vi "Test LoadCell200K_MBDC API.vi"() -> ()   [LabVIEW 2016]
doc: "LoadCell200K_MBDC API Tester."
uses:
  LoadCell200K_MBDC.lvlib
panel:
  in  "wait for reply":bool=TRUE
  in  "Show Block Diagram":bool
  in  "X":dbl=1.0
  out "Reply Payload":dbl
  in  "Stop Module":bool
  in  "Start Module":bool
  out "Do Something Count":i32
  in  "Test Do Something Else and Wait for Reply":bool
  in  "Hide Module Panel":bool
  in  "Show Module Panel":bool
  in  "Test Do Something Else":bool
  in  "Test Do Something":bool
  out "Status":string
  out "Module Running?":bool
  # "This VI tests the API for the Module."
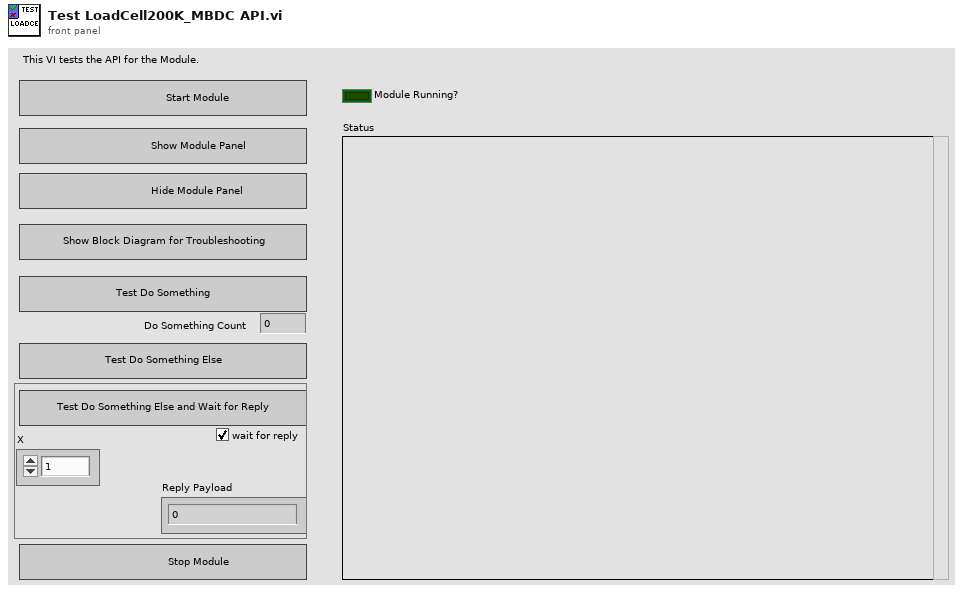
[diagram p1: front panel]
types:
  T1 = typedef "LoadCell200K_MBDC.lvlib/Broadcast Events--cluster.ctl" = cluster{"Module Did Init":refnum<user-event>, "Status Updated":refnum<user-event>, "Error Reported":refnum<user-event>, "Did Something":refnum<user-event>, "Module Did Stop":refnum<user-event>, "Update Module Execution Status":refnum<user-event>}
  T2 = typedef "LoadCell200K_MBDC.lvlib/Do Something Else and Wait (Reply Payload)--cluster.ctl" = cluster{"Value":dbl, "error":errorcluster}
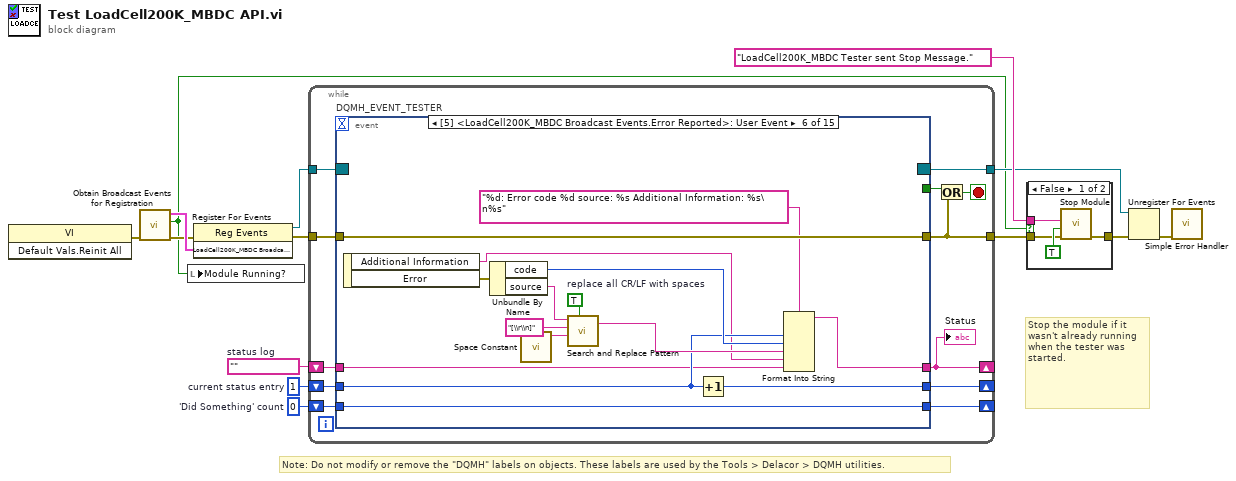
[diagram p0: block diagram]
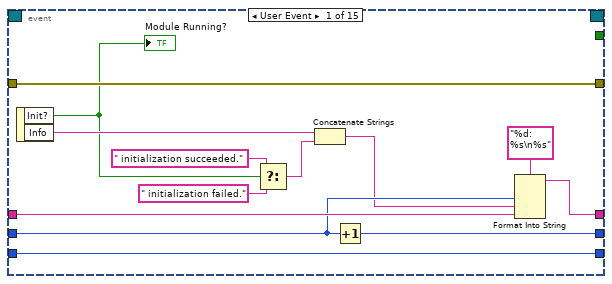
[diagram p3: hidden frame]
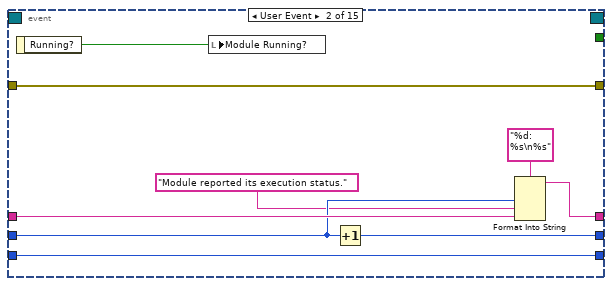
[diagram p4: hidden frame]
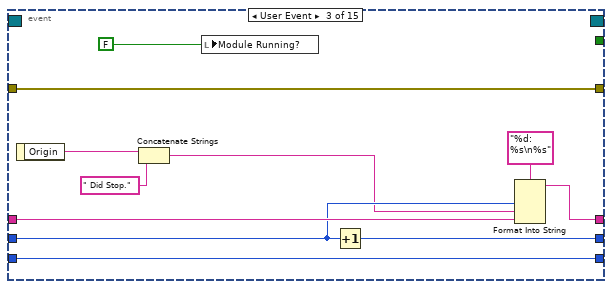
[diagram p5: hidden frame]
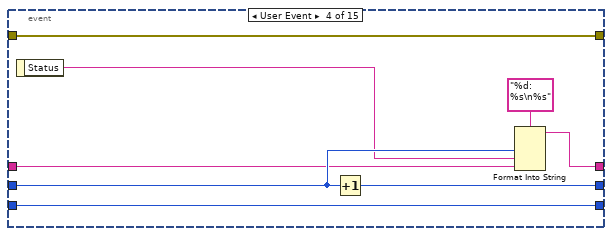
[diagram p6: hidden frame]
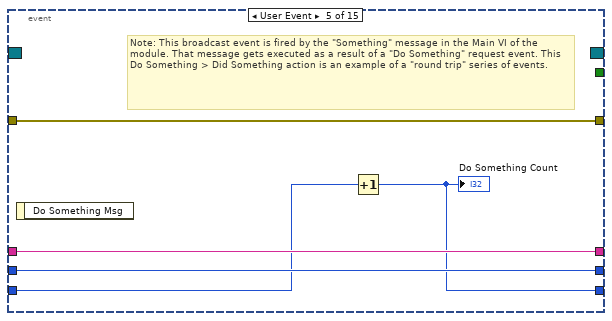
[diagram p7: hidden frame]
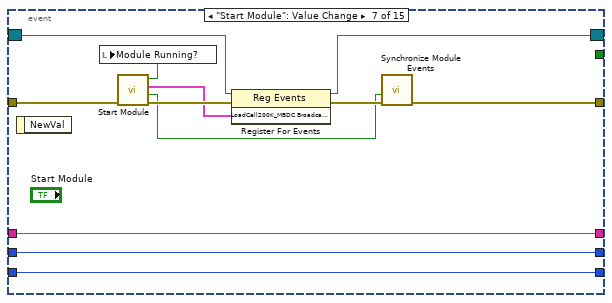
[diagram p8: hidden frame]
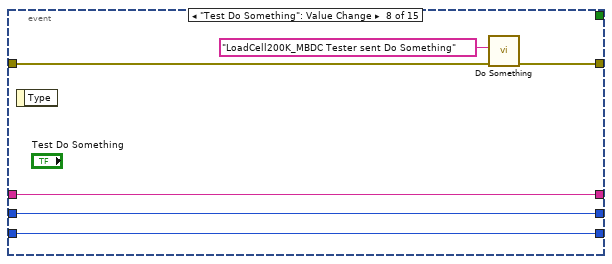
[diagram p9: hidden frame]
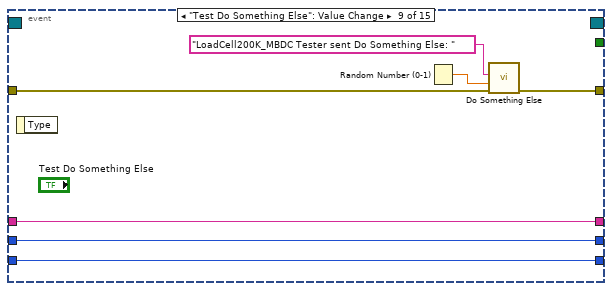
[diagram p10: hidden frame]
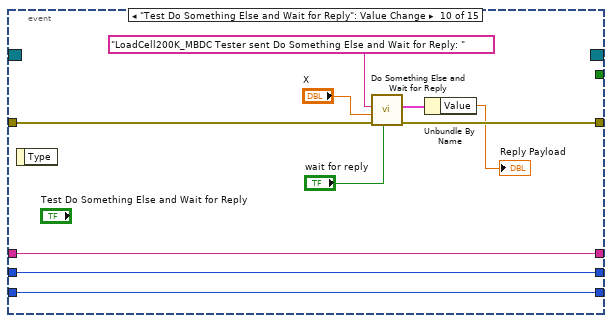
[diagram p11: hidden frame]
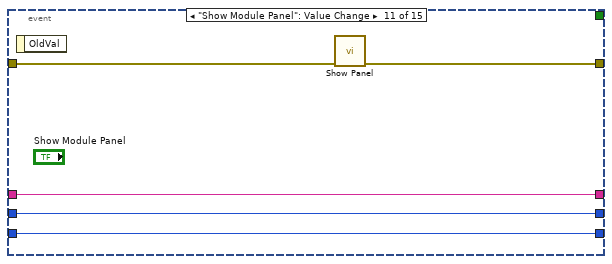
[diagram p12: hidden frame]
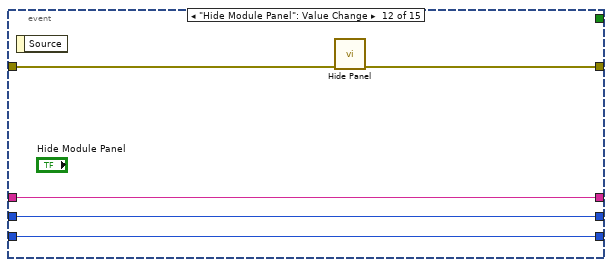
[diagram p13: hidden frame]
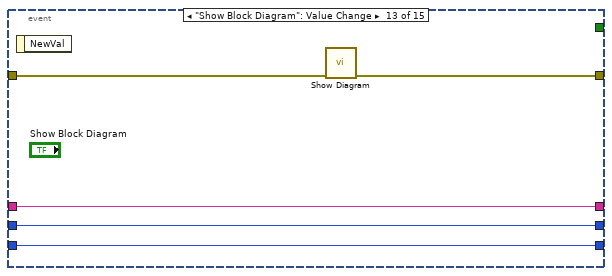
[diagram p14: hidden frame]
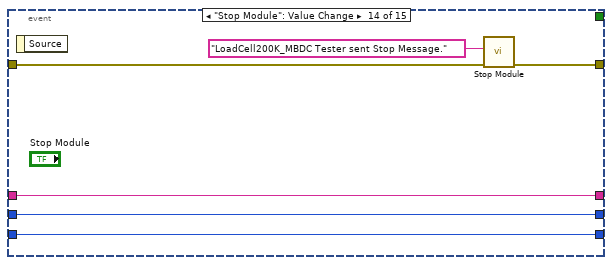
[diagram p15: hidden frame]
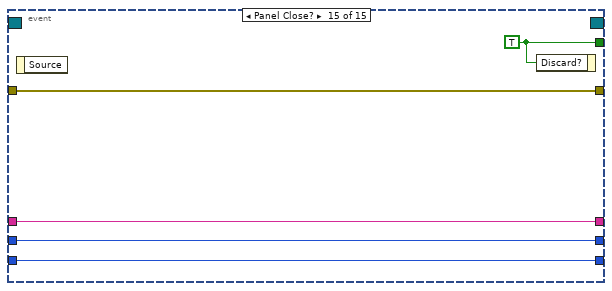
[diagram p16: hidden frame]
diagram:
  w10 = 0  # 'Did Something' count
  w11 = 1  # current status entry
  w12 = ""  # status log
  # "Stop the module if it wasn't already running when the tester was started."
  # "Note: Do not modify or remove the \"DQMH\" labels on objects. These labels are used by the Tools > Delacor > DQMH utilities."
  n1 = invoke class="VI" method="Default Vals.Reinit All"() -> (error out=w5:errorcluster)  [unwired: 3 in, 2 out]
  n2 = call "Obtain Broadcast Events for Registration.vi"("error in (no error)"=w5) -> ("error out"=w4:errorcluster, "Already running?"=w3:bool, "LoadCell200K_MBDC Broadcast Events"=w8:T1)  [unwired: 8 in]
  n3 = local write "Module Running?"(w3) -> ()
  n4 = register-events(error in=w4, w8) -> (reference out=w7:refnum<event-registration>, error out=w9:errorcluster)  [unwired: 1 in]
  n5 = while {
    tunnel: w7 -> [w26]
    tunnel: [w15] -> w2
    shift-right: [w21] -> _
    shift-left: w12 -> [w23]
    shift-right: [w22] -> _
    shift-left: w11 -> [w24]
    shift-right: [w19] -> _
    shift-left: w10 -> [w20]
    tunnel: w9 -> [w17]
    tunnel: [w16] -> w6
    stop <- w18 stop-if-true
    n6 = event "DQMH_EVENT_TESTER" shown="[5] <LoadCell200K_MBDC Broadcast Events.Error Reported>: User Event" {
      selector: w26 -> [_ _ _ _ _ _ w92 _ _ _ _ _ _ _ _]
      dyn-events: [_ _ _ _ _ _ w91 _ _ _ _ _ _ _ _] -> w16
      timeout: _ -> [_ _ _ _ _ _ _ _ _ _ _ _ _ _ _]
      tunnel: [_ _ _ _ _ _ _ _ _ _ _ _ _ _ w148] -> w25
      tunnel: [w39 w41 w49 w60 w68 w86 w90 w105 w112 w122 w127 w132 w133 w140 w144] -> w15
      tunnel: w24 -> [w36 w46 w57 w64 w71 w76 w96 w102 w108 w119 w125 w130 w135 w142 w146]
      tunnel: w23 -> [w37 w47 w58 w63 w72 w74 w97 w103 w109 w120 w126 w131 w136 w143 w147]
      tunnel: [w34 w44 w55 w65 w72 w77 w97 w103 w109 w120 w126 w131 w136 w143 w147] -> w21
      tunnel: [w35 w45 w56 w67 w71 w75 w96 w102 w108 w119 w125 w130 w135 w142 w146] -> w22
      tunnel: w20 -> [w31 w42 w51 w61 w70 w87 w95 w101 w107 w118 w124 w129 w134 w141 w145]
      tunnel: [w31 w42 w51 w61 w69 w87 w95 w101 w107 w118 w124 w129 w134 w141 w145] -> w19
      tunnel: w17 -> [w39 w41 w49 w60 w68 w86 w89 w100 w106 w115 w123 w128 w137 w138 w144]
      event User Event {
        n7 = event-data() -> ("Init?"=w30:bool, "Info"=w33:string)  [unwired: 1 in]
        "Module Running?" <- w30
        n8 = Select(t=" initialization succeeded.", s=w30, f=" initialization failed.") -> (s? t:f=w27:string)
        n9 = Concatenate Strings(w33, w27) -> (w32:string)
        n10 = Increment(x=w36) -> (x+1=w35:i32)
        n11 = Format Into String(format string="%d: %s\n%s", w36, w32, w37) -> (resulting string=w34:string)  [unwired: 2 in, 1 out]
      }
      event User Event {
        n12 = event-data() -> ("Running?"=w40:bool)  [unwired: 1 in]
        n13 = local write "Module Running?"(w40) -> ()
        n14 = Increment(x=w46) -> (x+1=w45:i32)
        n15 = Format Into String(format string="%d: %s\n%s", w46, "Module reported its execution status.", w47) -> (resulting string=w44:string)  [unwired: 2 in, 1 out]
      }
      event User Event {
        n16 = event-data() -> ("Origin"=w54:string)  [unwired: 1 in]
        n17 = Concatenate Strings(w54, " Did Stop.") -> (w53:string)
        n18 = local write "Module Running?"(FALSE ("Module Did Init?")) -> ()
        n19 = Increment(x=w57) -> (x+1=w56:i32)
        n20 = Format Into String(format string="%d: %s\n%s", w57, w53, w58) -> (resulting string=w55:string)  [unwired: 2 in, 1 out]
      }
      event User Event {
        n21 = event-data() -> ("Status"=w62:string)  [unwired: 1 in]
        n22 = Increment(x=w64) -> (x+1=w67:i32)
        n23 = Format Into String(format string="%d: %s\n%s", w64, w62, w63) -> (resulting string=w65:string)  [unwired: 2 in, 1 out]
      }
      event User Event {
        # "Note: This broadcast event is fired by the \"Something\" message in the Main VI of the module. That message gets executed as a result of a \"Do Something\" request event. This Do Something > Did Something action is an example of a \"round trip\" series of events."
        n24 = event-data() -> ()  [unwired: 1 in, 1 out]
        n25 = Increment(x=w70) -> (x+1=w69:i32)
        "Do Something Count" <- w69
      }
      event User Event {
        w82 = TRUE  # replace all CR/LF with spaces
        n26 = event-data() -> ("Additional Information"=w73:string, "Error"=w78:errorcluster)  [unwired: 1 in]
        n27 = Unbundle By Name(w78) -> ("code"=w79:i32, "source"=w80:string)
        n28 = call <vilib>:"Space Constant.vi"() -> ("String"=w83:string)
        n29 = call <vilib>:"Search and Replace Pattern.vi"("string"=w80, "regular expression (\"\")"="[\\r\\n]" ("regular expression (\"\")"), "replace string (\"\")"=w83, "replace all? (F)"=w82) -> ("result string"=w81:string)  [unwired: 1 in, 1 out]
        n30 = Increment(x=w76) -> (x+1=w75:i32)
        n31 = Format Into String(format string="%d: Error code %d source: %s Additional Information: %s\n%s", w76, w79, w81, w73, w74) -> (resulting string=w77:string)  [unwired: 2 in, 1 out]
      }
      event "Start Module": Value Change {
        n32 = event-data() -> ()  [unwired: 1 in, 1 out]
        n33 = call "Start Module.vi"("error in (no error)"=w89) -> ("error out"=w98:errorcluster, "Wait for Event Sync?"=w94:bool, "LoadCell200K_MBDC Broadcast Events"=w93:T1, "Module Was Already Running?"=w88:bool)  [unwired: 7 in]
        n34 = local write "Module Running?"(w88) -> ()
        n35 = register-events(reference=w92, error in=w98, w93) -> (reference out=w91:refnum<event-registration>, error out=w99:errorcluster)
        n36 = call "Synchronize Module Events.vi"("error in"=w99, "Wait for Event Sync?"=w94) -> ("error out"=w90:errorcluster)  [unwired: 9 in]
      }
      event "Test Do Something": Value Change {
        n37 = event-data() -> ()  [unwired: 1 in, 1 out]
        n38 = call "Do Something.vi"("error in (no error)"=w100, "Do Something Message"="LoadCell200K_MBDC Tester sent Do Something") -> ("error out"=w105:errorcluster)  [unwired: 9 in]
      }
      event "Test Do Something Else": Value Change {
        n39 = event-data() -> ()  [unwired: 1 in, 1 out]
        n40 = Random Number (0-1)() -> (number: 0 to 1=w110:dbl)
        n41 = call "Do Something Else.vi"("error in (no error)"=w106, "X"=w110, "Do Something Else Message"="LoadCell200K_MBDC Tester sent Do Something Else: " ("Do Something Message")) -> ("error out"=w112:errorcluster)  [unwired: 8 in]
      }
      event "Test Do Something Else and Wait for Reply": Value Change {
        n42 = event-data() -> ()  [unwired: 1 in, 1 out]
        n43 = call "Do Something Else and Wait for Reply.vi"("wait for reply (T)"="wait for reply", "error in (no error)"=w115, "X"="X", "Do Something Else Message"="LoadCell200K_MBDC Tester sent Do Something Else and Wait for Reply: " ("Do Something Message")) -> ("error out"=w122:errorcluster, "Reply Payload"=w117:T2)  [unwired: 5 in, 1 out]
        n44 = Unbundle By Name(w117) -> ("Value"=→"Reply Payload":dbl)
      }
      event "Show Module Panel": Value Change {
        n45 = event-data() -> ()  [unwired: 1 in, 1 out]
        n46 = call "Show Panel.vi"("error in (no error)"=w123) -> ("error out"=w127:errorcluster)  [unwired: 10 in]
      }
      event "Hide Module Panel": Value Change {
        n47 = event-data() -> ()  [unwired: 1 in, 1 out]
        n48 = call "Hide Panel.vi"("error in (no error)"=w128) -> ("error out"=w132:errorcluster)  [unwired: 10 in]
      }
      event "Show Block Diagram": Value Change {
        n49 = event-data() -> ()  [unwired: 1 in, 1 out]
        n50 = call "Show Diagram.vi"("error in (no error)"=w137) -> ("error out"=w133:errorcluster)  [unwired: 10 in]
      }
      event "Stop Module": Value Change {
        n51 = event-data() -> ()  [unwired: 1 in, 1 out]
        n52 = call "Stop Module.vi"("error in"=w138, "Origin"="LoadCell200K_MBDC Tester sent Stop Message.") -> ("error out"=w140:errorcluster)  [unwired: 9 in]
      }
      event Panel Close? {
        w148 = TRUE ("Discard?")
        n53 = event-data() -> ()  [unwired: 1 in, 1 out]
        n54 = event-data("Discard?"=w148) -> ()  [unwired: 1 in, 1 out]
      }
    }
    "Status" <- w21
    n55 = Or(x=w25, y=w15) -> (x .or. y?=w18:bool)
  }
  n56 = case shown="False" w3 {
    tunnel: [w152 w153] -> w14
    tunnel: "LoadCell200K_MBDC Tester sent Stop Message." ("Origin") -> [w151 _]
    tunnel: w2 -> [w149 w153]
    frame False {
      n57 = call "Stop Module.vi"("error in"=w149, "Wait for Module to Stop? (F)"=TRUE ("Wait for Module to stop?"), "Origin"=w151) -> ("error out"=w152:errorcluster)  [unwired: 8 in]
    }
    frame True {
    }
  }
  n58 = Unregister For Events(event registration refnum=w6, error in=w14) -> (error out=w1:errorcluster)
  n59 = call <vilib>:"Simple Error Handler.vi"("error in (no error)"=w1) -> ()  [unwired: 4 in, 5 out]
